vi "Configurate Coordenates.vi"(8 "Error In":errorcluster, 10 "Coordenates":T1 {"Longitude" format="%#_13g"; "Latitude" format="%#_13g"}, 11 "Open Weather Session In":refnum<class "Open Weather Session.lvclass">) -> (0 "Error Out":errorcluster, 3 "Open Weather Session Out":refnum<class "Open Weather Session.lvclass">)   [LabVIEW 2019, in "Open Weather Session.lvclass"]
uses:
  Open Weather Session.lvclass
  Controls/Coordenates.ctl
  Accessors/Coordenates/Set Coordenates.vi
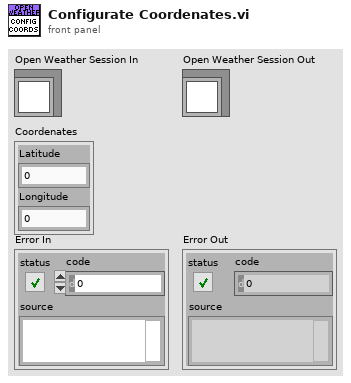
[diagram p1: front panel]
types:
  T1 = typedef "Open Weather Session.lvclass/Coordenates.ctl" = cluster{"Latitude":dbl, "Longitude":dbl}
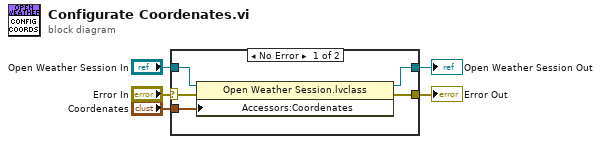
[diagram p0: block diagram]
diagram:
  n1 = case shown="No Error" "Error In" {
    selector: "Error In" -> [w10 w11]
    tunnel: [w8 w11] -> w4
    tunnel: [w7 w12] -> w3
    tunnel: "Open Weather Session In" -> [w9 w12]
    tunnel: "Coordenates" -> [w6 _]
    frame No Error {
      n2 = property class="Open Weather Session.lvclass"(reference=w9, error in=w10, "Accessors:Coordenates"=w6) -> (reference out=w7:refnum<class "Open Weather Session.lvclass">, error out=w8:errorcluster)
    }
    frame Error {
    }
  }
  "Error Out" <- w4
  "Open Weather Session Out" <- w3
